vi "SubVI_EXA bandwith_sweep.vi"(0 "VISA Refnum in":refnum<visa-resource-name>, 1 "Enable Continuous Sweep Mode (F: Disable)":bool, 2 "Enable Auto Sweep Time (T: Enable)":bool=TRUE, 3 "Enable Auto Resolution BandWidth (T: Enable)":bool=TRUE, 5 "Manual Sweep Time (265 ms)":dbl=0.265, 7 "Enable Auto Video BandWidth (T: Enable)":bool=TRUE, 9 "Manual Resolution BandWidth (3 MHz)":dbl=50880.0, 11 "error in (no error)":errorcluster, 12 "RBW Unit":u16(ring) items=["Hz", "KHz", "MHz"], 13 "Manual Video BandWidth (3 MHz)":dbl=-14656.0, 14 "VBW Unit":u16(ring) items=["Hz", "KHz", "MHz"]) -> (4 "VISA resource name":refnum<visa-resource-name>, 15 "error out":errorcluster)   [LabVIEW 2016]
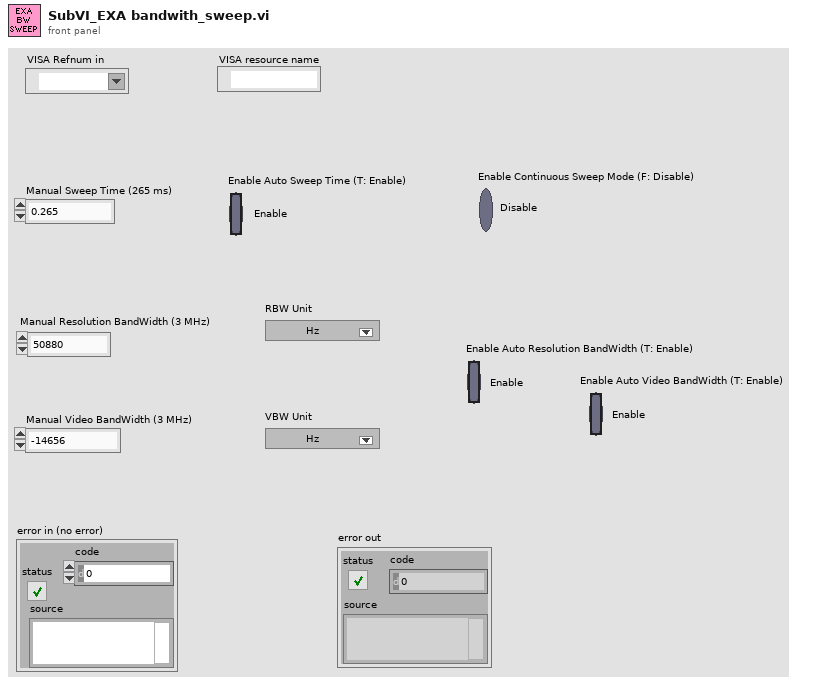
[diagram p1: front panel]
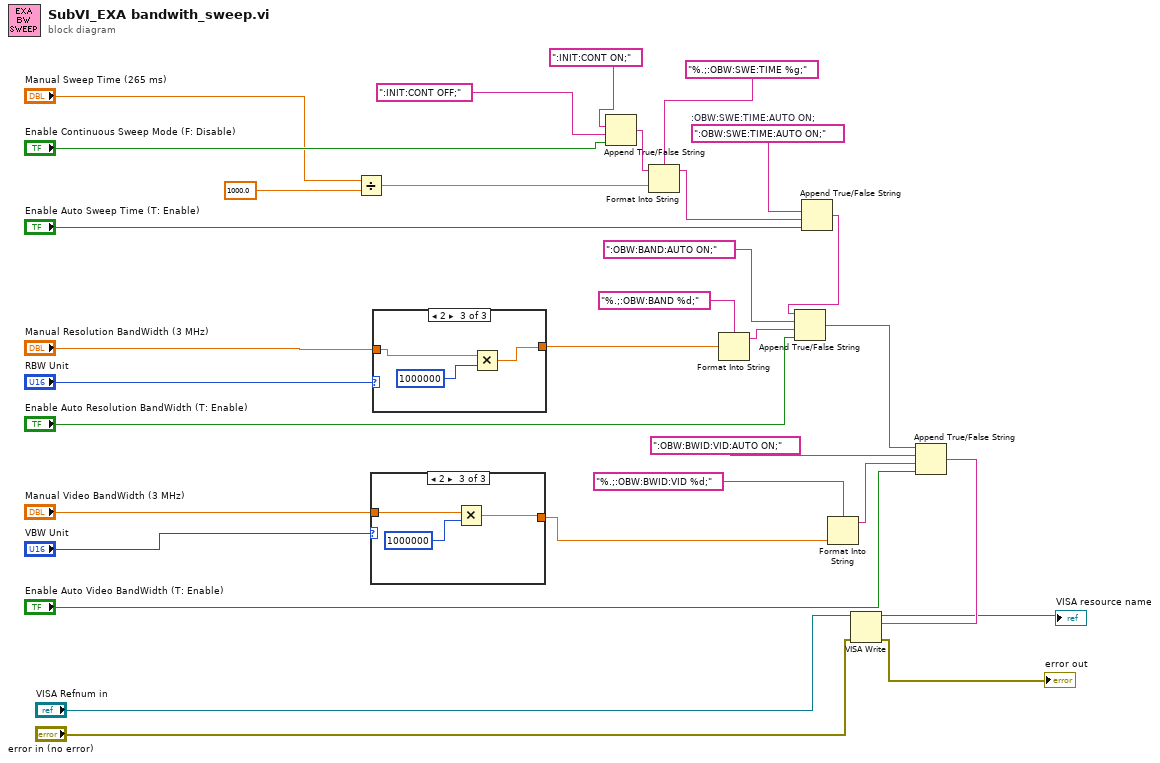
[diagram p0: block diagram]
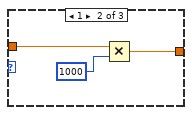
[diagram p3: hidden frame]
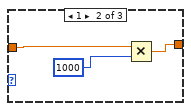
[diagram p5: hidden frame]
diagram:
  w4 = ":OBW:SWE:TIME:AUTO ON;"  # :OBW:SWE:TIME:AUTO ON;
  n1 = Divide(x="Manual Sweep Time (265 ms)", y=1000.0) -> (x/y=w24:dbl)
  n2 = case shown="2" "VBW Unit" {
    tunnel: "Manual Video BandWidth (3 MHz)" -> [w33 w36 w38]
    tunnel: [w33 w34 w37] -> w21
    frame 0, Default {
    }
    frame 1 {
      n3 = Multiply(x=w36, y=1000) -> (x*y=w34:dbl)
    }
    frame 2 {
      n4 = Multiply(x=w38, y=u32 1000000) -> (x*y=w37:dbl)
    }
  }
  n5 = case shown="2" "RBW Unit" {
    tunnel: "Manual Resolution BandWidth (3 MHz)" -> [w40 w43 w45]
    tunnel: [w40 w41 w44] -> w19
    frame 0, Default {
    }
    frame 1 {
      n6 = Multiply(x=w43, y=1000) -> (x*y=w41:dbl)
    }
    frame 2 {
      n7 = Multiply(x=w45, y=u32 1000000) -> (x*y=w44:dbl)
    }
  }
  n8 = Append True/False String(1:"Enable Continuous Sweep Mode (F: Disable)", 2:":INIT:CONT OFF;" ("string (\"\")"), 3:":INIT:CONT ON;" ("string (\"\")")) -> (0:w30:string)  [unwired: 1 in]
  n9 = Format Into String(format string="%.;:OBW:SWE:TIME %g;", initial string=w30, w24) -> (resulting string=w5:string)  [unwired: 1 in, 1 out]
  n10 = Format Into String(format string="%.;:OBW:BAND %d;", w19) -> (resulting string=w11:string)  [unwired: 2 in, 1 out]
  n11 = Append True/False String(1:"Enable Auto Sweep Time (T: Enable)", 2:w5, 3:w4) -> (0:w8:string)  [unwired: 1 in]
  n12 = Append True/False String(1:"Enable Auto Resolution BandWidth (T: Enable)", 2:w11, 3:":OBW:BAND:AUTO ON;" ("true string"), 4:w8) -> (0:w15:string)
  n13 = Format Into String(format string="%.;:OBW:BWID:VID %d;", w21) -> (resulting string=w13:string)  [unwired: 2 in, 1 out]
  n14 = Append True/False String(1:"Enable Auto Video BandWidth (T: Enable)", 2:w13, 3:":OBW:BWID:VID:AUTO ON;" ("true string"), 4:w15) -> (0:w26:string)
  n15 = VISA Write(VISA resource name="VISA Refnum in", write buffer=w26, error in (no error)="error in (no error)") -> (VISA resource name out=→"VISA resource name":refnum<visa-resource-name>, error out=→"error out":errorcluster)  [unwired: 1 out]
